vi "JSONtoControlValueCore.vi"(8 "error in":errorcluster, 10 "Value":T1, 11 "Control in":refnum<vi>) -> (0 "error out":errorcluster, 1 "Variant":variant)   [LabVIEW 2021]
uses:
  3bbbae6a-3930-4252-b221-5fb704abe217.vi
  4f307724-74bb-49c9-87fb-05fc31e080d8.vi
  5c9ce110-a408-4126-a7c2-1adb9af7b32e.vi
  8b0e1fe8-3f73-4a53-89fc-6f61fb9001f6.vi
  <vilib>/Comparison/Equal/Equal Functor/Equal Functor.lvclass
  <vilib>/regexp/Match Regular Expression.xnode
  <vilib>/Utility/Data Type/NI_Data Type.lvlib
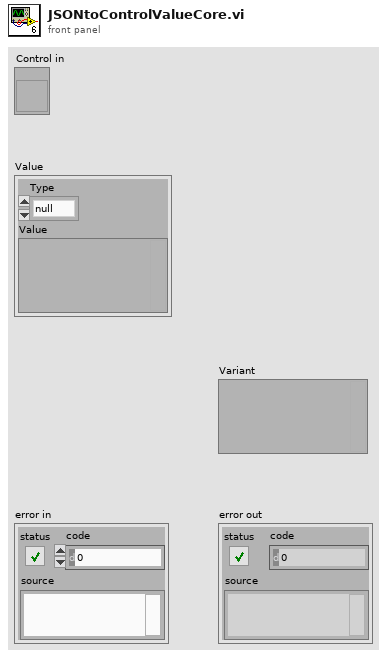
[diagram p1: front panel]
types:
  T1 = cluster{"Type":enum16{"null", "number", "boolean", "string", "array", "object", ""}, "Value":variant}
  T2 = enum16{"null", "number", "boolean", "string", "array", "object", ""}
  T3 = cluster{"Type":enum16{"null", "number", "boolean", "string", "array", "object", ""}, "Value":variant}[]
  T4 = typedef "LVStringsAndValuesArrayTypeDef.ctl" = cluster{"String":string, "Value":ext}[]
  T5 = map{string, cluster{"Type":enum16{"null", "number", "boolean", "string", "array", "object", ""}, "Value":variant}}
  T6 = typedef "NI_Data Type.lvlib/Refnum Type.ctl" = enum16{"NotARefnum", "UnknownRefnum", "Generic", "Datalog", "ByteStream", "Device", "Occurence", "TCPNetConnection", "Auto", "Menu", "Imaq", "Hardware", "DataSocket", "Visa", "IVI", "UDPNetConnection", "Notifier", "Queue", "Irda", "EventReg", "DotNet", "UserEvent", "Callback", "UNUSED_EMPTY_POSITION", "BlueToothNetConnection", "LVObjApp", "LVObjVI", "LVObjUnknown", "GenericClass", "UserDefinedRefnumTag", "DataValue", "RT FIFO", "TDMS File", "PythonSessionRefnum"}
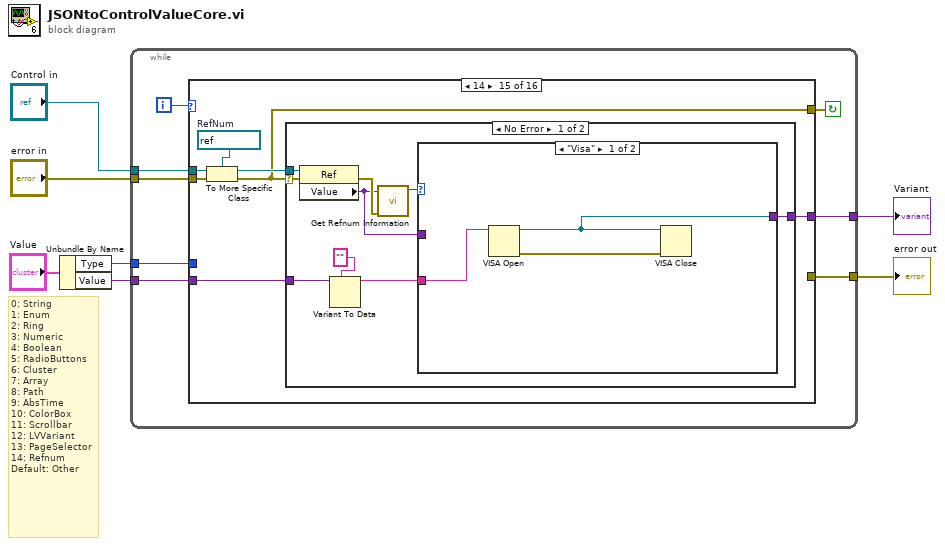
[diagram p0: block diagram]
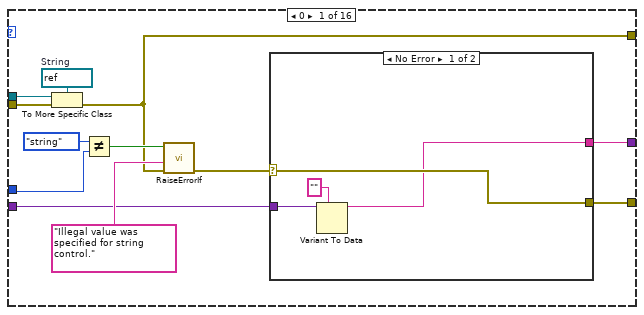
[diagram p2: hidden frame]
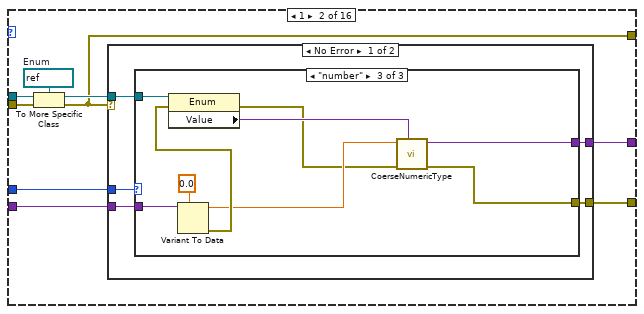
[diagram p4: hidden frame]
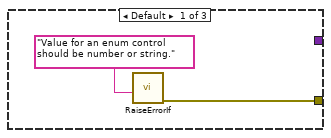
[diagram p5: hidden frame]
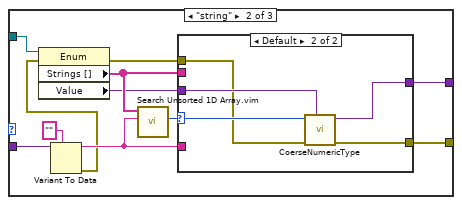
[diagram p6: hidden frame]
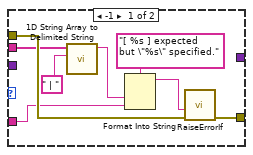
[diagram p7: hidden frame]
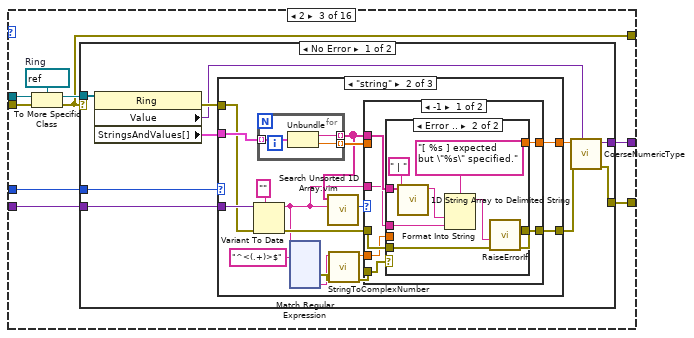
[diagram p9: hidden frame]
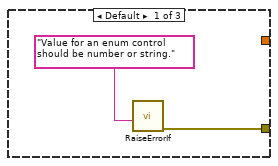
[diagram p10: hidden frame]
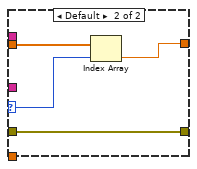
[diagram p12: hidden frame]
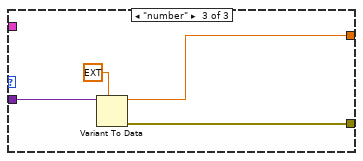
[diagram p13: hidden frame]
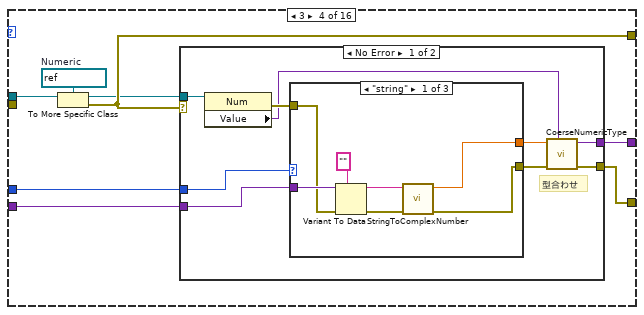
[diagram p15: hidden frame]
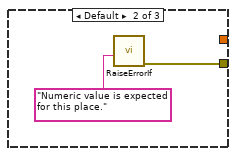
[diagram p16: hidden frame]
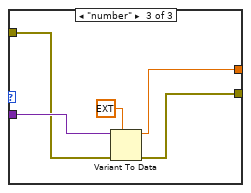
[diagram p17: hidden frame]
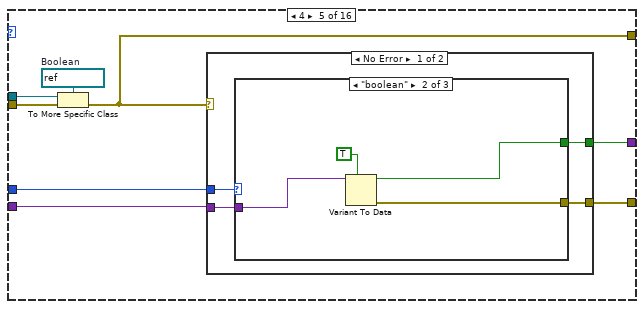
[diagram p19: hidden frame]
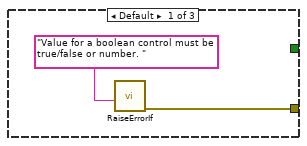
[diagram p20: hidden frame]
diagram:
  # "0: String\n1: Enum\n2: Ring\n3: Numeric\n4: Boolean\n5: RadioButtons\n6: Cluster\n7: Array\n8: Path\n9: AbsTime\n10: ColorBox\n11: Scrollbar\n12: LVVariant\n13: PageSelector\n14: Refnum\nDefault: Other"
  n1 = Unbundle By Name("Value") -> ("Type"=w3:T2, "Value"=w1:variant)
  n2 = while {
    tunnel: "Control in" -> [w14]
    tunnel: "error in" -> [w12]
    tunnel: [w13] -> w7
    tunnel: [w11] -> w5
    tunnel: w1 -> [w10]
    tunnel: w3 -> [w9]
    i -> [w15]
    stop <- w8 continue-if-true
    n3 = case shown="14" w15 {
      tunnel: w14 -> [w26 w40 w89 w271 w302 w326 w375 w434 w455 w469 w496 w517 w546 w555 w599 w618]
      tunnel: [w20 w37 w86 w269 w301 w323 w370 w430 w452 w467 w494 w515 w545 w553 w595 errorcluster {"status"=FALSE, "code"=0, "source"=""} ("error out")] -> w8
      tunnel: [w17 w39 w83 w270 w298 w325 w374 w432 w454 w468 w495 w516 w542 w554 w596 _] -> w13
      tunnel: w12 -> [w25 w36 w87 _ w296 w322 _ _ w453 _ _ _ _ _ w600 _]
      tunnel: [w18 w35 w82 w266 w297 w321 w372 w431 w447 w464 w491 w512 _ w550 _ w614] -> w11
      tunnel: w10 -> [w16 w33 w84 w268 w300 w319 w369 w424 w445 w465 w492 w514 w544 w551 w594 _]
      tunnel: w9 -> [w22 w34 w85 w267 w299 w320 w373 w426 w450 w466 w493 w513 w543 w552 _ _]
      frame 0 {
        w27 = refnum<vi> refnum  # String
        n4 = To More Specific Class(target class=w27, reference=w26, error in=w25) -> (error out=w20:errorcluster)  [unwired: 1 out]
        n5 = Not Equal?(x=T2."string" ("Type"), y=w22) -> (x != y?=w21:bool)
        n6 = call "RaiseErrorIf.vi"("error in (no error)"=w20, "error message"="Illegal value was specified for string control." ("error source (\" \")"), "error? (true)"=w21) -> ("error out"=w19:errorcluster)  [unwired: 8 in]
        n7 = case shown="No Error" w19 {
          selector: w19 -> [w31 w32]
          tunnel: [w31 w32] -> w18
          tunnel: [w28 _] -> w17
          tunnel: w16 -> [w30 _]
          frame No Error {
            n8 = Variant To Data(type="" ("delimiter"), Variant=w30) -> (data=w28:string)  [unwired: 1 in, 1 out]
          }
          frame Error {
          }
        }
      }
      frame 1 {
        w41 = refnum<vi> refnum  # Enum
        n9 = To More Specific Class(target class=w41, reference=w40, error in=w36) -> (specific class reference=w38:refnum<vi>, error out=w37:errorcluster)
        n10 = case shown="No Error" w37 {
          tunnel: [w46 _] -> w39
          tunnel: w38 -> [w45 _]
          tunnel: [w44 _] -> w35
          tunnel: w34 -> [w43 _]
          tunnel: w33 -> [w42 _]
          frame No Error {
            n11 = case shown="\"number\"" w43 {
              tunnel: [_ w59 w75] -> w46
              tunnel: w45 -> [_ w58 w79]
              tunnel: [w47 w55 w73] -> w44
              tunnel: w42 -> [_ w52 w81]
              frame Default {
                n12 = call "RaiseErrorIf.vi"("error message"="Value for an enum control  should be number or string." ("error source (\" \")")) -> ("error out"=w47:errorcluster)  [unwired: 10 in]
              }
              frame "string" {
                n13 = Variant To Data(type="", Variant=w52) -> (data=w51:string, error out=w50:errorcluster)  [unwired: 1 in]
                n14 = property class="Enum"(reference=w58, error in=w50) -> (error out=w56:errorcluster, "Strings []"=w54:string[], "Value"=w49:variant)  [unwired: 1 out]
                n15 = call "Search Unsorted 1D Array.vim"("element"=w51, "unsorted 1D array"=w54) -> ("index of element"=w57:i32)  [unwired: 9 in]
                n16 = case shown="Default" w57 {
                  selector: w57 -> [_ w71]
                  tunnel: [_ w72] -> w59
                  tunnel: w56 -> [w67 w69]
                  tunnel: w54 -> [w66 _]
                  tunnel: [w61 w68] -> w55
                  tunnel: w51 -> [w60 _]
                  tunnel: w49 -> [_ w70]
                  frame -1 {
                    n17 = call <vilib>:"1D String Array to Delimited String.vi"("delimiter"=" | ", "string array"=w66) -> ("delimited string"=w63:string)  [unwired: 9 in]
                    n18 = Format Into String(format string="[ %s ] expected but \"%s\" specified.", w63, w60) -> (resulting string=w62:string)  [unwired: 2 in, 1 out]
                    n19 = call "RaiseErrorIf.vi"("error in (no error)"=w67, "error message"=w62) -> ("error out"=w61:errorcluster)  [unwired: 9 in]
                  }
                  frame Default {
                    n20 = call "CoerseNumericType.vi"("Numeric Variant in"=w70, "error in (no error)"=w69, "Numeric"=w71) -> ("error out"=w68:errorcluster, "Numeric Variant out"=w72:variant)  [unwired: 7 in]
                  }
                }
              }
              frame "number" {
                n21 = Variant To Data(type=0.0, Variant=w81) -> (data=w77:dbl, error out=w78:errorcluster)  [unwired: 1 in]
                n22 = property class="Enum"(reference=w79, error in=w78) -> (error out=w74:errorcluster, "Value"=w76:variant)  [unwired: 1 out]
                n23 = call "CoerseNumericType.vi"("Numeric Variant in"=w76, "error in (no error)"=w74, "Numeric"=w77) -> ("error out"=w73:errorcluster, "Numeric Variant out"=w75:variant)  [unwired: 7 in]
              }
            }
          }
          frame Error {
          }
        }
      }
      frame 2 {
        w90 = refnum<vi> refnum  # Ring
        n24 = To More Specific Class(target class=w90, reference=w89, error in=w87) -> (specific class reference=w88:refnum<vi>, error out=w86:errorcluster)
        n25 = case shown="No Error" w86 {
          tunnel: w88 -> [w97 _]
          tunnel: [w93 _] -> w82
          tunnel: w85 -> [w100 _]
          tunnel: w84 -> [w99 _]
          tunnel: [w95 _] -> w83
          frame No Error {
            n26 = property class="Ring"(reference=w97) -> (error out=w98:errorcluster, "Value"=w91:variant, "StringsAndValues[]"=w92:T4)  [unwired: 1 in, 1 out]
            n27 = case shown="\"string\"" w100 {
              tunnel: [_ w118 w262] -> w96
              tunnel: [w101 w115 w261] -> w94
              tunnel: w99 -> [_ w114 w264]
              tunnel: w92 -> [_ w112 _]
              tunnel: w98 -> [_ w110 _]
              frame Default {
                n28 = call "RaiseErrorIf.vi"("error message"="Value for an enum control  should be number or string." ("error source (\" \")")) -> ("error out"=w101:errorcluster)  [unwired: 10 in]
              }
              frame "string" {
                n29 = Variant To Data(error in=w110, type="" ("delimiter"), Variant=w114) -> (data=w107:string, error out=w109:errorcluster)
                n30 = for {
                  tunnel: w112 -> [w240] mode=indexing
                  tunnel: [w239] -> w111 mode=indexing
                  tunnel: [w238] -> w116 mode=indexing
                  n31 = Unbundle(w240) -> ("String"=w239:string, "Value"=w238:ext)
                }
                n32 = xnode "Match Regular Expression"("input string"=w107, "regular expression"="^<(.+)>$") -> ("error out"=w106:errorcluster, "submatch 1"=w105:string)  [unwired: 4 in, 4 out]
                n33 = call "Search Unsorted 1D Array.vim"("element"=w107, "unsorted 1D array"=w111) -> ("index of element"=w117:i32)  [unwired: 9 in]
                n34 = call "StringToComplexNumber.vi"("error in (no error)"=w106, "input string"=w105) -> ("error out"=w104:errorcluster, "x + iy"=w103:cxt)  [unwired: 8 in]
                n35 = case shown="-1" w117 {
                  selector: w117 -> [_ w260]
                  tunnel: [w241 w258] -> w118
                  tunnel: w116 -> [_ w259]
                  tunnel: [w247 w257] -> w115
                  tunnel: w111 -> [w246 _]
                  tunnel: w107 -> [w245 _]
                  tunnel: w109 -> [w244 w257]
                  tunnel: w104 -> [w243 _]
                  tunnel: w103 -> [w242 _]
                  frame -1 {
                    n36 = case shown="Error .." w243 {
                      tunnel: [_ w252] -> w247
                      tunnel: w246 -> [_ w251]
                      tunnel: w245 -> [_ w250]
                      tunnel: w244 -> [_ w249]
                      tunnel: w242 -> [w248 _]
                      tunnel: [w248 _] -> w241
                      frame No Error {
                      }
                      frame Error {
                        n37 = call <vilib>:"1D String Array to Delimited String.vi"("delimiter"=" | ", "string array"=w251) -> ("delimited string"=w254:string)  [unwired: 9 in]
                        n38 = Format Into String(format string="[ %s ] expected but \"%s\" specified.", w254, w250) -> (resulting string=w253:string)  [unwired: 2 in, 1 out]
                        n39 = call "RaiseErrorIf.vi"("error in (no error)"=w249, "error message"=w253) -> ("error out"=w252:errorcluster)  [unwired: 9 in]
                      }
                    }
                  }
                  frame Default {
                    n40 = Index Array(array=w259, index=w260) -> (element=w258:ext)
                  }
                }
              }
              frame "number" {
                n41 = Variant To Data(type=ext 0.0, Variant=w264) -> (data=w262:ext, error out=w261:errorcluster)  [unwired: 1 in]
              }
            }
            n42 = call "CoerseNumericType.vi"("Numeric Variant in"=w91, "error in (no error)"=w94, "Numeric"=w96) -> ("error out"=w93:errorcluster, "Numeric Variant out"=w95:variant)  [unwired: 7 in]
          }
          frame Error {
          }
        }
      }
      frame 3 {
        w272 = refnum<vi> refnum  # Numeric
        n43 = To More Specific Class(target class=w272, reference=w271) -> (specific class reference=w265:refnum<vi>, error out=w269:errorcluster)  [unwired: 1 in]
        n44 = case shown="No Error" w269 {
          tunnel: [w273 _] -> w270
          tunnel: w268 -> [w281 _]
          tunnel: w267 -> [w280 _]
          tunnel: [w274 _] -> w266
          tunnel: w265 -> [w279 _]
          frame No Error {
            # "型合わせ"
            n45 = property class="Num"(reference=w279) -> (error out=w278:errorcluster, "Value"=w277:variant)  [unwired: 1 in, 1 out]
            n46 = case shown="\"string\"" w280 {
              tunnel: w281 -> [w288 _ w295]
              tunnel: w278 -> [w285 _ w293]
              tunnel: [w283 w289 w292] -> w276
              tunnel: [w282 _ w291] -> w275
              frame "string" {
                n47 = Variant To Data(error in=w285, type="", Variant=w288) -> (data=w286:string, error out=w284:errorcluster)
                n48 = call "StringToComplexNumber.vi"("error in (no error)"=w284, "input string"=w286) -> ("error out"=w283:errorcluster, "x + iy"=w282:cxt)  [unwired: 8 in]
              }
              frame Default {
                n49 = call "RaiseErrorIf.vi"("error message"="Numeric value is expected for this place." ("error source (\" \")")) -> ("error out"=w289:errorcluster)  [unwired: 10 in]
              }
              frame "number" {
                n50 = Variant To Data(error in=w293, type=ext 0.0 ("number"), Variant=w295) -> (data=w291:ext, error out=w292:errorcluster)
              }
            }
            n51 = call "CoerseNumericType.vi"("Numeric Variant in"=w277, "error in (no error)"=w276, "Numeric"=w275) -> ("error out"=w274:errorcluster, "Numeric Variant out"=w273:variant)  [unwired: 7 in]
          }
          frame Error {
          }
        }
      }
      frame 4 {
        w303 = refnum<vi> refnum  # Boolean
        n52 = To More Specific Class(target class=w303, reference=w302, error in=w296) -> (error out=w301:errorcluster)  [unwired: 1 out]
        n53 = case shown="No Error" w301 {
          tunnel: w299 -> [w307 _]
          tunnel: w300 -> [w306 _]
          tunnel: [w305 _] -> w298
          tunnel: [w304 _] -> w297
          frame No Error {
            n54 = case shown="\"boolean\"" w307 {
              tunnel: w306 -> [_ w313 w317]
              tunnel: [_ w311 w318] -> w305
              tunnel: [w309 w310 w314] -> w304
              frame Default {
                n55 = call "RaiseErrorIf.vi"("error message"="Value for a boolean control must be true/false or number. " ("error source (\" \")")) -> ("error out"=w309:errorcluster)  [unwired: 10 in]
              }
              frame "boolean" {
                n56 = Variant To Data(type=TRUE, Variant=w313) -> (data=w311:bool, error out=w310:errorcluster)  [unwired: 1 in]
              }
              frame "number" {
                n57 = Variant To Data(type=ext 0.0, Variant=w317) -> (data=w315:ext, error out=w314:errorcluster)  [unwired: 1 in]
                n58 = Not Equal To 0?(x=w315) -> (x != 0?=w318:bool)
              }
            }
          }
          frame Error {
          }
        }
      }
      frame 5 {
        w327 = refnum<vi> refnum  # RadioButtonsControl
        n59 = To More Specific Class(target class=w327, reference=w326, error in=w322) -> (specific class reference=w324:refnum<vi>, error out=w323:errorcluster)
        n60 = case shown="No Error" w323 {
          tunnel: [w332 _] -> w325
          tunnel: w324 -> [w331 _]
          tunnel: [w330 _] -> w321
          tunnel: w320 -> [w329 _]
          tunnel: w319 -> [w328 _]
          frame No Error {
            n61 = case shown="\"string\"" w329 {
              tunnel: [_ w346 w362] -> w332
              tunnel: w331 -> [_ w345 w366]
              tunnel: [w333 w343 w360] -> w330
              tunnel: w328 -> [_ w341 w368]
              frame Default {
                n62 = call "RaiseErrorIf.vi"("error message"="Value for an enum control  should be number or string." ("error source (\" \")")) -> ("error out"=w333:errorcluster)  [unwired: 10 in]
              }
              frame "string" {
                n63 = Variant To Data(type="", Variant=w341) -> (data=w337:string, error out=w340:errorcluster)  [unwired: 1 in]
                n64 = property class="RadioBtnsControl"(reference=w345, error in=w340) -> (error out=w338:errorcluster, "Value"=w339:variant)  [unwired: 1 out]
                n65 = call <vilib>:"Get Numeric Information.vi"("error in (no error)"=w338, "variant"=w339) -> ("error out"=w336:errorcluster, "enum names"=w335:string[])  [unwired: 6 in, 2 out]
                n66 = call "Search Unsorted 1D Array.vim"("element"=w337, "unsorted 1D array"=w335) -> ("index of element"=w344:i32)  [unwired: 9 in]
                n67 = case shown="-1" w344 {
                  selector: w344 -> [_ w358]
                  tunnel: [_ w359] -> w346
                  tunnel: w336 -> [w354 w356]
                  tunnel: [w349 w355] -> w343
                  tunnel: w337 -> [w348 _]
                  tunnel: w339 -> [_ w357]
                  tunnel: w335 -> [w347 _]
                  frame -1 {
                    n68 = call <vilib>:"1D String Array to Delimited String.vi"("delimiter"=" | ", "string array"=w347) -> ("delimited string"=w351:string)  [unwired: 9 in]
                    n69 = Format Into String(format string="[ %s ] expected but \"%s\" specified.", w351, w348) -> (resulting string=w350:string)  [unwired: 2 in, 1 out]
                    n70 = call "RaiseErrorIf.vi"("error in (no error)"=w354, "error message"=w350) -> ("error out"=w349:errorcluster)  [unwired: 9 in]
                  }
                  frame Default {
                    n71 = call "CoerseNumericType.vi"("Numeric Variant in"=w357, "error in (no error)"=w356, "Numeric"=w358) -> ("error out"=w355:errorcluster, "Numeric Variant out"=w359:variant)  [unwired: 7 in]
                  }
                }
              }
              frame "number" {
                n72 = Variant To Data(type=0.0, Variant=w368) -> (data=w364:dbl, error out=w365:errorcluster)  [unwired: 1 in]
                n73 = property class="RadioBtnsControl"(reference=w366, error in=w365) -> (error out=w361:errorcluster, "Value"=w363:variant)  [unwired: 1 out]
                n74 = call "CoerseNumericType.vi"("Numeric Variant in"=w363, "error in (no error)"=w361, "Numeric"=w364) -> ("error out"=w360:errorcluster, "Numeric Variant out"=w362:variant)  [unwired: 7 in]
              }
            }
          }
          frame Error {
          }
        }
      }
      frame 6 {
        w376 = refnum<vi> refnum  # Cluster
        n75 = To More Specific Class(target class=w376, reference=w375) -> (specific class reference=w371:refnum<vi>, error out=w370:errorcluster)  [unwired: 1 in]
        n76 = case shown="No Error" w370 {
          tunnel: [w385 _] -> w374
          tunnel: w373 -> [w381 _]
          tunnel: [w386 _] -> w372
          tunnel: w371 -> [w384 _]
          tunnel: w369 -> [w380 _]
          frame No Error {
            n77 = property class="Clust"(reference=w384) -> (error out=w377:errorcluster, "Value"=w383:variant, "Controls[]"=w382:refnum<vi>[])  [unwired: 1 in, 1 out]
            n78 = call "JSONObjectToMap.vi"("error in"=w377, "Value"=w380, "Type"=w381) -> ("error out"=w379:errorcluster, "Map"=w378:T5)  [unwired: 7 in]
            n79 = call <vilib>:"Get Cluster Information.vi"("error in (no error)"=w379, "variant"=w383) -> ("error out"=w390:errorcluster, "cluster elements"=w391:variant[])  [unwired: 8 in]
            n80 = Variant To Flattened String(Variant=w383) -> (data string=w392:string, 1:w388:i16[])
            n81 = for {
              shift-right: [w407] -> _
              shift-left: w392 -> [w406]
              tunnel: w391 -> [w416] mode=indexing
              tunnel: w382 -> [w405] mode=indexing
              shift-right: [w403] -> w387
              shift-left: w390 -> [w414]
              tunnel: [w411] -> w389 mode=concatenating
              tunnel: w378 -> [w399]
              i -> [w401]
              n82 = Number To Decimal String(number=w401) -> (decimal integer string=w400:string)  [unwired: 1 in]
              n83 = Variant To Flattened String(Variant=w416) -> (1:w415:i16[])  [unwired: 1 out]
              n84 = call <vilib>:"Get Type Information.vi"("error in (no error)"=w414, "variant"=w416) -> ("error out"=w413:errorcluster, "name"=w402:string)  [unwired: 5 in, 3 out]
              n85 = Look In Map(map=w399, key=w402) -> (key not found?=w396:bool, value=w398:T1)  [unwired: 1 in]
              n86 = Look In Map(map=w399, key=w400) -> (key not found?=w395:bool, value=w397:T1)  [unwired: 1 in]
              n87 = Flattened String To Variant(4:w413, 6:w406, 7:w415) -> (0:w404:errorcluster, 3:w410:variant)
              n88 = And(x=w396, y=w395) -> (x .and. y?=w394:bool)
              n89 = Select(t=w397, s=w396, f=w398) -> (s? t:f=w393:T1)
              n90 = case shown="False" w394 {
                tunnel: w410 -> [_ w423]
                tunnel: [w420 w423] -> w412
                tunnel: w405 -> [w421 _]
                tunnel: w404 -> [w419 w422]
                tunnel: [w418 w422] -> w403
                tunnel: w393 -> [w417 _]
                frame False {
                  n91 = call "JSONtoControlValueCore.vi"("error in"=w419, "Value"=w417, "Control in"=w421) -> ("error out"=w418:errorcluster, "Variant"=w420:variant)  [unwired: 7 in]
                }
                frame True {
                }
              }
              n92 = Variant To Flattened String(Variant=w410) -> (data string=w409:string)  [unwired: 1 out]
              n93 = String Length(string=w409) -> (length=w408:i32)
              n94 = String Subset(string=w406, offset (0)=w408) -> (substring=w407:string)  [unwired: 1 in]
              n95 = Variant To Flattened String(Variant=w412) -> (data string=w411:string)  [unwired: 1 out]
            }
            n96 = Flattened String To Variant(4:w387, 6:w389, 7:w388) -> (0:w386:errorcluster, 3:w385:variant)
          }
          frame Error {
          }
        }
      }
      frame 7 {
        w435 = refnum<vi> refnum  # Array
        n97 = To More Specific Class(target class=w435, reference=w434) -> (specific class reference=w433:refnum<vi>, error out=w430:errorcluster)  [unwired: 1 in]
        n98 = Not Equal?(x=T2."array" ("Type"), y=w426) -> (x != y?=w428:bool)
        n99 = call "RaiseErrorIf.vi"("error in (no error)"=w430, "error message"="Illegal value was specified for an array." ("error source (\" \")"), "error? (true)"=w428) -> ("error out"=w429:errorcluster)  [unwired: 8 in]
        n100 = case shown="No Error" w429 {
          selector: w429 -> [w440 w444]
          tunnel: w433 -> [w442 _]
          tunnel: [w439 variant[] []] -> w432
          tunnel: [w441 w444] -> w431
          tunnel: w424 -> [w437 _]
          frame No Error {
            n101 = Variant To Data(type=T3 [], Variant=w437) -> (data=w436:T3)  [unwired: 1 in, 1 out]
            n102 = call "JSONtoArrayValue.vi"("error in (no error)"=w440, "data (parsed JSON)"=w436, "Array in"=w442) -> ("error out"=w441:errorcluster, "Variant"=w439:variant)  [unwired: 7 in]
          }
          frame Error {
          }
        }
      }
      frame 8 {
        w456 = refnum<vi> refnum  # Path
        n103 = To More Specific Class(target class=w456, reference=w455, error in=w453) -> (error out=w452:errorcluster)  [unwired: 1 out]
        n104 = Not Equal?(x=T2."string" ("Type"), y=w450) -> (x != y?=w449:bool)
        n105 = call "RaiseErrorIf.vi"("error message"="Path value should be string." ("error source (\" \")"), "error? (true)"=w449) -> ("error out"=w448:errorcluster)  [unwired: 9 in]
        n106 = case shown="No Error" w452 {
          tunnel: [w463 _] -> w454
          tunnel: w448 -> [w458 _]
          tunnel: [w457 _] -> w447
          tunnel: w445 -> [w461 _]
          frame No Error {
            n107 = Variant To Data(error in=w458, type="", Variant=w461) -> (data=w459:string, error out=w457:errorcluster)
            n108 = String To Path(string=w459) -> (path=w462:path)
            n109 = To Variant(anything=w462) -> (Variant=w463:variant)
          }
          frame Error {
          }
        }
      }
      frame 9 {
        w470 = refnum<vi> refnum  # AbsTime
        n110 = To More Specific Class(target class=w470, reference=w469) -> (error out=w467:errorcluster)  [unwired: 1 in, 1 out]
        n111 = case shown="No Error" w467 {
          tunnel: [w474 _] -> w468
          tunnel: w466 -> [w473 _]
          tunnel: w465 -> [w472 _]
          tunnel: [w471 _] -> w464
          frame No Error {
            n112 = case shown="\"string\"" w473 {
              tunnel: [_ w487] -> w474
              tunnel: w472 -> [_ w486]
              tunnel: [w475 w478] -> w471
              frame Default {
                n113 = call "RaiseErrorIf.vi"("error message"="AbsTime value should be specified by string." ("error source (\" \")")) -> ("error out"=w475:errorcluster)  [unwired: 10 in]
              }
              frame "string" {
                n114 = Variant To Data(type="" ("delimiter"), Variant=w486) -> (data=w484:string, error out=w483:errorcluster)  [unwired: 1 in]
                n115 = Scan From String(format string="%T", input string=w484, error in=w483) -> (remaining string=w481:string, error out=w479:errorcluster, output 1=w488:timestamp)  [unwired: 2 in, 1 out]
                n116 = Not Equal?(x="", y=w481) -> (x != y?=w480:bool)
                n117 = call "RaiseErrorIf.vi"("error in (no error)"=w479, "error message"="Specified value can not be interpreted as time.", "error? (true)"=w480) -> ("error out"=w478:errorcluster)  [unwired: 8 in]
                n118 = To Variant(anything=w488) -> (Variant=w487:variant)
              }
            }
          }
          frame Error {
          }
        }
      }
      frame 10 {
        w497 = refnum<vi> refnum  # ColorBox
        n119 = To More Specific Class(target class=w497, reference=w496) -> (specific class reference=w490:refnum<vi>, error out=w494:errorcluster)  [unwired: 1 in]
        n120 = case shown="No Error" w494 {
          tunnel: [w502 _] -> w495
          tunnel: w493 -> [w501 _]
          tunnel: w492 -> [w500 _]
          tunnel: [w499 _] -> w491
          tunnel: w490 -> [w498 _]
          frame No Error {
            n121 = case shown="\"number\"" w501 {
              tunnel: [_ w510] -> w502
              tunnel: w500 -> [_ w509]
              tunnel: [w504 w507] -> w499
              tunnel: w498 -> [_ w506]
              frame Default {
                n122 = call "RaiseErrorIf.vi"("error message"="Color Box value should be specified by number." ("error source (\" \")")) -> ("error out"=w504:errorcluster)  [unwired: 10 in]
              }
              frame "number" {
                # "U32"
                n123 = property class="ColBox"(reference=w506) -> ("Value"=w505:u32)  [unwired: 1 in, 2 out]
                n124 = Variant To Data(type=w505, Variant=w509) -> (data=w508:u32, error out=w507:errorcluster)  [unwired: 1 in]
                n125 = To Variant(anything=w508) -> (Variant=w510:variant)
              }
            }
          }
          frame Error {
          }
        }
      }
      frame 11 {
        w518 = refnum<vi> refnum  # Scrollbar
        n126 = To More Specific Class(target class=w518, reference=w517) -> (specific class reference=w511:refnum<vi>, error out=w515:errorcluster)  [unwired: 1 in]
        n127 = case shown="No Error" w515 {
          tunnel: [w519 _] -> w516
          tunnel: w514 -> [w527 _]
          tunnel: w513 -> [w526 _]
          tunnel: [w520 _] -> w512
          tunnel: w511 -> [w525 _]
          frame No Error {
            # "型合わせ"
            n128 = property class="Scroll"(reference=w525) -> (error out=w524:errorcluster, "Value"=w523:variant)  [unwired: 1 in, 1 out]
            n129 = case shown="\"string\"" w526 {
              tunnel: w527 -> [w534 _ w541]
              tunnel: w524 -> [w531 _ w539]
              tunnel: [w529 w535 w538] -> w522
              tunnel: [w528 _ w537] -> w521
              frame "string" {
                n130 = Variant To Data(error in=w531, type="", Variant=w534) -> (data=w532:string, error out=w530:errorcluster)
                n131 = call "StringToComplexNumber.vi"("error in (no error)"=w530, "input string"=w532) -> ("error out"=w529:errorcluster, "x + iy"=w528:cxt)  [unwired: 8 in]
              }
              frame Default {
                n132 = call "RaiseErrorIf.vi"("error message"="Numeric value is expected for this place." ("error source (\" \")")) -> ("error out"=w535:errorcluster)  [unwired: 10 in]
              }
              frame "number" {
                n133 = Variant To Data(error in=w539, type=ext 0.0 ("number"), Variant=w541) -> (data=w537:ext, error out=w538:errorcluster)
              }
            }
            n134 = call "CoerseNumericType.vi"("Numeric Variant in"=w523, "error in (no error)"=w522, "Numeric"=w521) -> ("error out"=w520:errorcluster, "Numeric Variant out"=w519:variant)  [unwired: 7 in]
          }
          frame Error {
          }
        }
      }
      frame 12 {
        w547 = refnum<vi> refnum  # LVVariant
        n135 = To More Specific Class(target class=w547, reference=w546) -> (error out=w545:errorcluster)  [unwired: 1 in, 1 out]
        n136 = case shown="No Error" w545 {
          tunnel: w544 -> [w548 _]
          tunnel: w543 -> [_ _]
          tunnel: [w548 _] -> w542
          frame No Error {
          }
          frame Error {
          }
        }
      }
      frame 13 {
        w556 = refnum<vi> refnum  # PageSelector
        n137 = To More Specific Class(target class=w556, reference=w555) -> (specific class reference=w549:refnum<vi>, error out=w553:errorcluster)  [unwired: 1 in]
        n138 = case shown="No Error" w553 {
          tunnel: [w561 _] -> w554
          tunnel: w552 -> [w560 _]
          tunnel: w551 -> [w559 _]
          tunnel: [w558 _] -> w550
          tunnel: w549 -> [w557 _]
          frame No Error {
            n139 = case shown="\"string\"" w560 {
              tunnel: [_ w566 w580] -> w561
              tunnel: w559 -> [_ w571 w582]
              tunnel: [w563 w564 w578] -> w558
              tunnel: w557 -> [_ w570 w581]
              frame Default {
                n140 = call "RaiseErrorIf.vi"("error message"="PageSelector value should be specified by number." ("error source (\" \")")) -> ("error out"=w563:errorcluster)  [unwired: 10 in]
              }
              frame "number" {
                n141 = property class="PageSel"(reference=w570) -> ("Value"=w567:variant)  [unwired: 1 in, 2 out]
                n142 = Variant To Data(type=0, Variant=w571) -> (data=w568:i32, error out=w565:errorcluster)  [unwired: 1 in]
                n143 = call "CoerseNumericType.vi"("Numeric Variant in"=w567, "error in (no error)"=w565, "Numeric"=w568) -> ("error out"=w564:errorcluster, "Numeric Variant out"=w566:variant)  [unwired: 7 in]
              }
              frame "string" {
                # "ページ名\nを検索"
                n144 = Variant To Data(type="", Variant=w582) -> (data=w572:string, error out=w579:errorcluster)  [unwired: 1 in]
                n145 = property class="PageSel"(reference=w581) -> ("Value"=w574:variant, "Pages"=w576:refnum<vi>[])  [unwired: 1 in, 2 out]
                n146 = for {
                  tunnel: w576 -> [w593] mode=indexing
                  tunnel: [w592] -> w575 mode=indexing
                  n147 = property class="Page"(reference=w593) -> ("PageLabel"=w592:string)  [unwired: 1 in, 2 out]
                }
                n148 = call "Search Unsorted 1D Array.vim"("element"=w572, "unsorted 1D array"=w575) -> ("index of element"=w573:i32)  [unwired: 9 in]
                n149 = case shown="-1" w573 {
                  selector: w573 -> [_ w587]
                  tunnel: [_ w591] -> w580
                  tunnel: w579 -> [_ w590]
                  tunnel: [w586 w589] -> w578
                  tunnel: w574 -> [_ w588]
                  tunnel: w572 -> [w585 _]
                  frame -1 {
                    n150 = Concatenate Strings("Page not found: ", w585) -> (w584:string)
                    n151 = call "RaiseErrorIf.vi"("error message"=w584) -> ("error out"=w586:errorcluster)  [unwired: 10 in]
                  }
                  frame Default {
                    n152 = call "CoerseNumericType.vi"("Numeric Variant in"=w588, "error in (no error)"=w590, "Numeric"=w587) -> ("error out"=w589:errorcluster, "Numeric Variant out"=w591:variant)  [unwired: 7 in]
                  }
                }
              }
            }
          }
          frame Error {
          }
        }
      }
      frame 14 {
        w598 = refnum<vi> refnum  # RefNum
        n153 = To More Specific Class(target class=w598, reference=w599, error in=w600) -> (specific class reference=w597:refnum<vi>, error out=w595:errorcluster)
        n154 = case shown="No Error" w595 {
          selector: w595 -> [w606 _]
          tunnel: w597 -> [w609 _]
          tunnel: [w605 _] -> w596
          tunnel: w594 -> [w603 _]
          frame No Error {
            n155 = property class="Ref"(reference=w609, error in=w606) -> (error out=w608:errorcluster, "Value"=w604:variant)  [unwired: 1 out]
            n156 = Variant To Data(type="", Variant=w603) -> (data=w601:string)  [unwired: 1 in, 1 out]
            n157 = call <vilib>:"Get Refnum Information.vi"("error in (no error)"=w608, "variant"=w604) -> ("reference type"=w607:T6)  [unwired: 6 in, 3 out]
            n158 = case shown="\"Visa\"" w607 {
              tunnel: w601 -> [w612 _]
              tunnel: [w610 w613] -> w605
              tunnel: w604 -> [_ w613]
              frame "Visa" {
                n159 = VISA Open(VISA resource name=w612) -> (VISA resource name=w610:refnum<visa-resource-name>, error out=w611:errorcluster)  [unwired: 4 in]
                n160 = VISA Close(VISA resource name=w610, error in (no error)=w611) -> ()  [unwired: 1 out]
              }
              frame Default {
              }
            }
          }
          frame Error {
          }
        }
      }
      frame Default {
        # "stop"
        n161 = property class="Ctl"(reference=w618) -> ("ClassName"=w616:string)  [unwired: 1 in, 2 out]
        n162 = Format Into String(format string="Writing into \"%s\" is not supported.", w616) -> (resulting string=w615:string)  [unwired: 2 in, 1 out]
        n163 = call "RaiseErrorIf.vi"("error message"=w615) -> ("error out"=w614:errorcluster)  [unwired: 10 in]
      }
    }
  }
  "Variant" <- w7
  "error out" <- w5
